vi "Colour Ramp.vi"(9 "End colour":u32(colorbox)=6618880, 10 "Start colour":u32(colorbox)=16711680, 11 "No of colours":i32=10) -> (2 "Colour Array 2":u32[](array[colorbox]), 3 "Colour Array":u32[](array[numeric]))   [LabVIEW 2020]
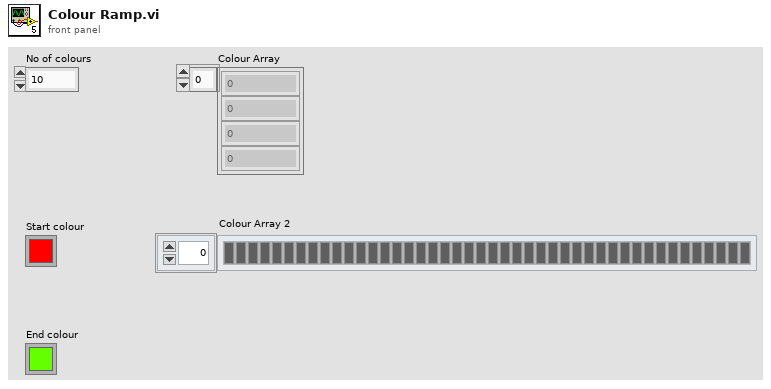
[diagram p1: front panel]
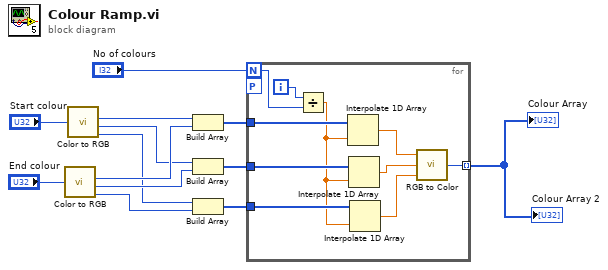
[diagram p0: block diagram]
diagram:
  n1 = call <vilib>:"Color to RGB.vi"("Color"="End colour") -> ("R"=w7:u8, "G"=w8:u8, "B"=w9:u8)  [unwired: 1 out]
  n2 = call <vilib>:"Color to RGB.vi"("Color"="Start colour") -> ("R"=w4:u8, "G"=w5:u8, "B"=w6:u8)  [unwired: 1 out]
  n3 = Build Array(w4, w7) -> (w10:u8[])
  n4 = Build Array(w5, w8) -> (w11:u8[])
  n5 = Build Array(w6, w9) -> (w12:u8[])
  n6 = for {
    N: "No of colours" -> [w14]
    tunnel: w10 -> [w23]
    tunnel: w11 -> [w22]
    tunnel: w12 -> [w21]
    tunnel: [w16] -> w13 mode=indexing
    workers-P: _ -> [_]
    i -> [w15]
    n7 = Divide(x=w15, y=w14) -> (x/y=w20:dbl)
    n8 = Interpolate 1D Array(1:w20, 2:w23) -> (0:w19:dbl)
    n9 = Interpolate 1D Array(1:w20, 2:w22) -> (0:w18:dbl)
    n10 = Interpolate 1D Array(1:w20, 2:w21) -> (0:w17:dbl)
    n11 = call <vilib>:"RGB to Color.vi"("B"=w17, "G"=w18, "R"=w19) -> ("Color"=w16:u32)
  }
  "Colour Array" <- w13
  "Colour Array 2" <- w13
